vi "group_by.vi"() -> ()   [LabVIEW 2017, in "tools.lvlib"]
uses:
  tools.lvlib
panel:
  out "Numeric":i32
  out "Array":cluster{"data OUT":dbl[][]}[](array[cluster])
  in  "column index":i32
  in  "data IN":dbl[][](array[numeric])
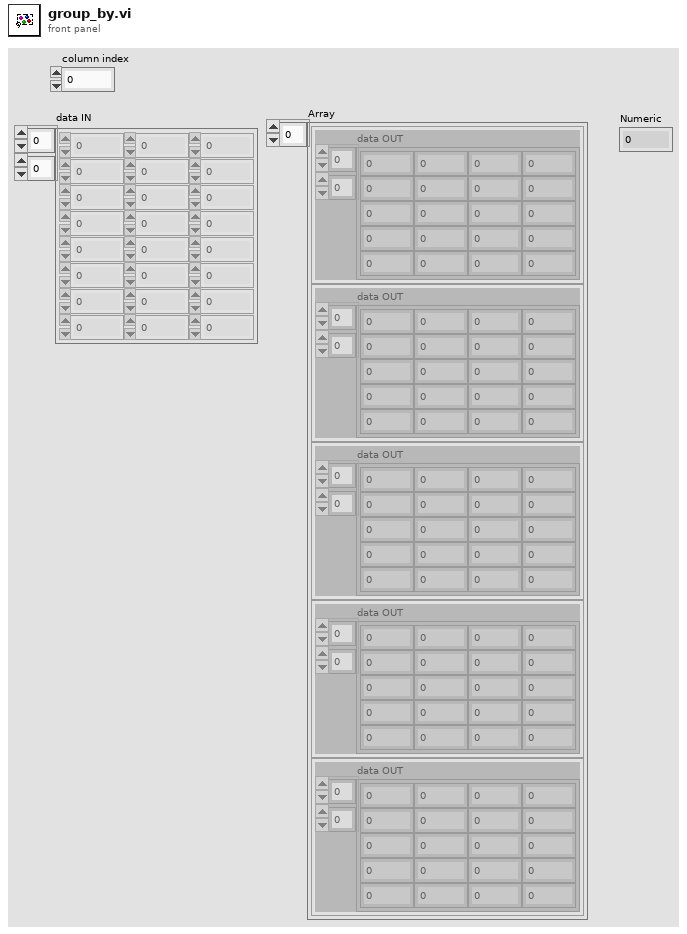
[diagram p1: front panel]
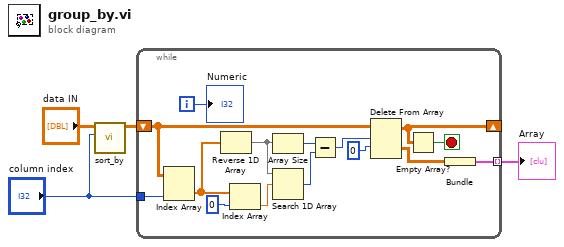
[diagram p0: block diagram]
diagram:
  n1 = call "sort_by.vi"("column index"="column index", "data IN"="data IN") -> ("data OUT"=w3:dbl[][])  [unwired: 9 in]
  n2 = while {
    shift-right: [w15] -> _
    shift-left: w3 -> [w18]
    tunnel: "column index" -> [w19]
    tunnel: [w16] -> w1 mode=indexing
    i -> [w13]
    stop <- w14 stop-if-true
    n3 = Index Array(array=w18, index (col)=w19) -> (element=w11:dbl[])  [unwired: 1 in]
    n4 = Reverse 1D Array(array=w11) -> (reversed array=w9:dbl[])
    n5 = Index Array(array=w11, index=0) -> (element=w10:dbl)
    n6 = Array Size(array=w9) -> (size(s)=w7:i32)
    n7 = Search 1D Array(1D array=w9, element=w10) -> (index of element=w6:i32)  [unwired: 1 in]
    n8 = Subtract(x=w7, y=w6) -> (x-y=w8:i32)
    n9 = Delete From Array(array=w18, length=w8, index (row)=0) -> (deleted portion=w17:dbl[][], array with subset deleted=w15:dbl[][])  [unwired: 1 in]
    n10 = Empty Array?(array=w15) -> (empty?=w14:bool)
    n11 = Bundle("data OUT"=w17) -> (w16:cluster{"data OUT":dbl[][]})  [unwired: 1 in]
    "Numeric" <- w13
  }
  "Array" <- w1
